vi "Is VI Reference WFP.vi"(8 "error in (no error)":errorcluster, 10 "VI Refnum":refnum<vi>, 11 "Web FP In":refnum<class "Web Front Panel.lvclass">) -> (0 "error out":errorcluster, 2 "VI Reference Is WFP":bool, 3 "Web FP Out":refnum<class "Web Front Panel.lvclass">)   [LabVIEW 2015, in "Front Panel Publisher.lvlib" / "Web Front Panel.lvclass"]
uses:
  Web Front Panel.lvclass
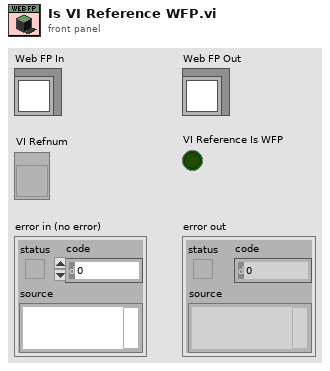
[diagram p1: front panel]
types:
  T1 = typedef "Front Panel Publisher.lvlib/Web Front Panel.lvclass/Object Attributes.ctl" = cluster{"VI Name":string, "VI Reference":refnum<vi>, "Controls":refnum<class "Object.lvclass">[], "Indicators":refnum<class "Object.lvclass">[], "Decorations":refnum<class "Object.lvclass">[], "VR With Previous Get":refnum<data-value>, "VR With Ring Images":refnum<data-value>}
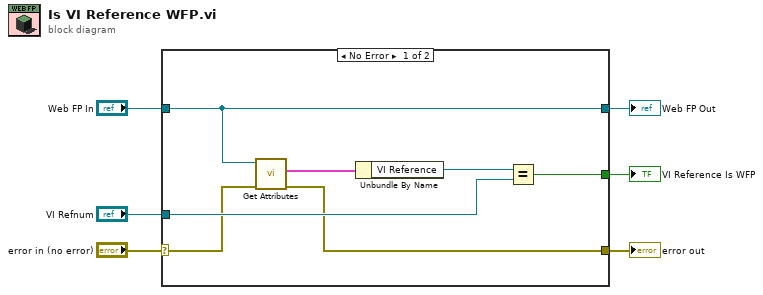
[diagram p0: block diagram]
diagram:
  n1 = case shown="No Error" "error in (no error)" {
    selector: "error in (no error)" -> [w8 w15]
    tunnel: [w7 w15] -> w5
    tunnel: [w13 w14] -> w3
    tunnel: "Web FP In" -> [w13 w14]
    tunnel: "VI Refnum" -> [w11 _]
    tunnel: [w9 _] -> w1
    frame No Error {
      n2 = call "Get Attributes.vi"("error in (no error)"=w8, "Web FP In"=w13) -> ("error out"=w7:errorcluster, "Data"=w12:T1)  [unwired: 6 in, 2 out]
      n3 = Unbundle By Name(w12) -> ("VI Reference"=w10:refnum<vi>)
      n4 = Equal?(x=w10, y=w11) -> (x = y?=w9:bool)
    }
    frame Error {
    }
  }
  "error out" <- w5
  "Web FP Out" <- w3
  "VI Reference Is WFP" <- w1
